vi "GetMyRIOAccel.vi"(8 "error in (no error)":errorcluster) -> (0 "error out":errorcluster, 3 "output cluster":T1)   [LabVIEW 2017]
uses:
  <vilib>/myRIO/Instrument Drivers/Onboard Devices/Accelerometer/typedefs/Accelerometer Reference.ctl
  <vilib>/myRIO/Common/Instrument Driver Framework/Utilities/typedefs/myRIO Generic Hardware Reference.ctl
  <vilib>/myRIO/Common/Instrument Driver Framework/Utilities/typedefs/Hardware Version Enum.ctl
  <vilib>/myRIO/Common/Instrument Driver Framework/Utilities/typedefs/myRIO v1.0 Reference.ctl
  <vilib>/myRIO/Common/Instrument Driver Framework/Utilities/typedefs/Generic FPGA Reference.ctl
  <vilib>/myRIO/Common/Instrument Driver Framework/myRIO v1.0/Accelerometer/typedefs/Accelerometer Channels List.ctl
  <vilib>/myRIO/Common/Instrument Driver Framework/myRIO v1.0/Accelerometer/typedefs/Accelerometer Channels Enum.ctl
  <vilib>/userdefined/High Color/nirio_resource_hc.ctl
  <vilib>/myRIO/Common/Instrument Driver Framework/Utilities/vis/Is FPGA Ref Available.vi
  <vilib>/myRIO/Common/Instrument Driver Framework/myRIO v1.0/Accelerometer/vis/myRIO v1.1 Open Accelerometer.vi
  <vilib>/myRIO/Instrument Drivers/Onboard Devices/Accelerometer/vis/Read.vi
  <vilib>/myRIO/Common/Instrument Driver Framework/Utilities/vis/Validate Channels.vi
  <vilib>/myRIO/Common/Instrument Driver Framework/myRIO v1.0/Accelerometer/vis/myRIO v1.0 Reserve Accelerometer.vi
  <vilib>/myRIO/Common/Instrument Driver Framework/myRIO v1.0/Resource Manager/vis/myRIO v1.0 Reserve Channel List.vi
  <vilib>/myRIO/Common/Instrument Driver Framework/myRIO v1.0/Accelerometer/vis/myRIO v1.0 Build MUX Configuration Accelerometer.vi
  <vilib>/myRIO/Common/Instrument Driver Framework/myRIO v1.0/Resource Manager/vis/myRIO v1.0 Reserve Channel.vi
  <vilib>/myRIO/Common/Instrument Driver Framework/myRIO v1.0/Resource Manager/vis/myRIO v1.0 Unreserve Channel.vi
  <vilib>/myRIO/Common/Instrument Driver Framework/myRIO v1.0/Resource Manager/vis/myRIO v1.0 Build Mutex Name.vi
  <vilib>/Utility/VariantDataType/GetNumericInfo.vi
  <vilib>/Utility/error.llb/Error Cluster From Error Code.vi
  <vilib>/myRIO/Common/Instrument Driver Framework/myRIO v1.0/myRIO v1.1 Open.vi
  <vilib>/myRIO/Common/Instrument Driver Framework/myRIO v1.0/Accelerometer/vis/myRIO v1.0 Get Scaling Constant Accelerometer.vi
  <vilib>/myRIO/Common/Instrument Driver Framework/Utilities/vis/IO Manager.vi
  <vilib>/myRIO/Common/Instrument Driver Framework/Utilities/vis/Configuration Manager.vi
  <vilib>/myRIO/Common/Instrument Driver Framework/myRIO v1.0/myRIO v1.0 Close.vi
  <vilib>/myRIO/Common/Instrument Driver Framework/myRIO v1.0/Accelerometer/vis/myRIO v1.0 Read Accelerometer.vi
  <vilib>/myRIO/Express VI/Onboard Devices/Accelerometer/Accelerometer Express VI.xnode
  <vilib>/myRIO/Instrument Drivers/Onboard Devices/Accelerometer/vis/myRIO Accelerometer Open.xnode
  <vilib>/myRIO/Instrument Drivers/Onboard Devices/Accelerometer/Accelerometer.lvlib
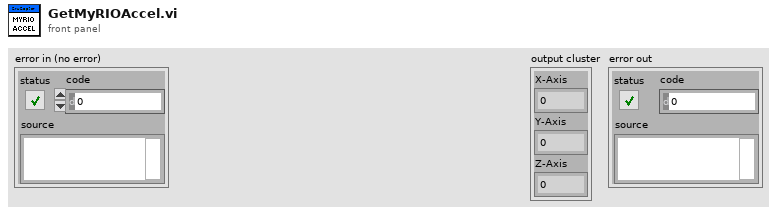
[diagram p1: front panel]
types:
  T1 = cluster{"X-Axis":dbl, "Y-Axis":dbl, "Z-Axis":dbl}
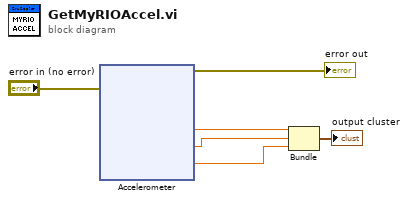
[diagram p0: block diagram]
diagram:
  n1 = xnode "Accelerometer"("error in (no error)"="error in (no error)") -> ("X-Axis"=w6:dbl, "Y-Axis"=w5:dbl, "Z-Axis"=w4:dbl, "error out"=→"error out":errorcluster)
  n2 = Bundle("X-Axis"=w6, "Y-Axis"=w5, "Z-Axis"=w4) -> (→"output cluster":T1)  [unwired: 1 in]
